vi "speed-test.vi"() -> ()   [LabVIEW 2020]
uses:
  <vilib>/Utility/Data Type/Type Definitions/Data Type.ctl
  <vilib>/Utility/Data Type/NI_Data Type.lvlib
panel:
  out "x-y":dbl
  out "Name":string
  out "number of dimensions":i32
  out "type":T1
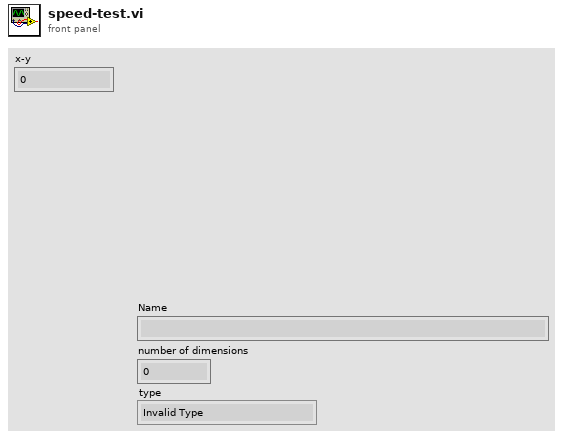
[diagram p1: front panel]
types:
  T1 = typedef "NI_Data Type.lvlib/Data Type.ctl" = enum8{"Invalid Type", "Void", "I8", "I16", "I32", "I64", "U8", "U16", "U32", "U64", "Single Float", "Double Float", "Extended Float", "Single Complex", "Double Complex", "Extended Complex", "Enum U8", "Enum U16", "Enum U32", "Enum U64", "Single Float With Unit", "Double Float With Unit", "Extended Float With Unit", "Single Complex with Unit", "Double Complex with Unit", "Extended Complex with Unit", "Boolean", "String", "Path", "Picture", "Tag", "Array", "Cluster", "Variant", "LV Variant", "Waveform", "Timestamp", "Digital Waveform", "Digital Data", "ExpressData", "Refnum", "External Data", "VI", "Poly VI", "LabVIEW Class Instance", "Fixed Point", "Set Collection", "Map Collection"}
  T2 = typedef "NI_Data Type.lvlib/Type Definition Info.ctl" = cluster{"Name":string, "Timestamp":u32}
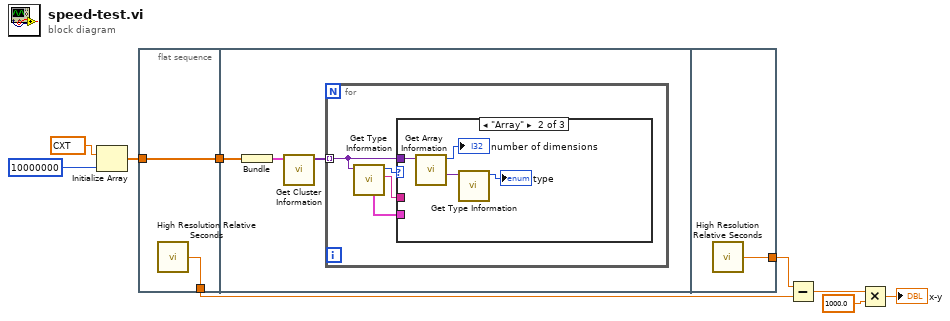
[diagram p0: block diagram]
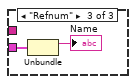
[diagram p3: hidden frame]
diagram:
  n1 = Initialize Array(cxt 0.0+0.0i ("element"), 10000000 ("dimension size")) -> (w7:cxt[])
  n2 = flat-sequence {
    tunnel: w7 -> [w11]
    tunnel: [w11] -> w6
    tunnel: [w10] -> w4
    tunnel: w6 -> [w13]
    tunnel: [w25] -> w5
    frame #0 {
      n3 = call <vilib>:"High Resolution Relative Seconds.vi"() -> ("relative seconds"=w10:dbl)
    }
    frame #1 {
      n4 = Bundle(w13) -> (w12:cluster{cxt[]})  [unwired: 1 in]
      n5 = call <vilib>:"Get Cluster Information.vi"("variant"=w12) -> ("cluster elements"=w14:variant[])  [unwired: 9 in, 1 out]
      n6 = for {
        tunnel: w14 -> [w15] mode=indexing
        n7 = call <vilib>:"Get Type Information.vi"("variant"=w15) -> ("name"=w16:string, "type"=w17:T1, "type definition info"=w18:T2)  [unwired: 6 in, 2 out]
        n8 = case shown="\"Array\"" w17 {
          tunnel: w18 -> [_ _ w24]
          tunnel: w16 -> [_ _ _]
          tunnel: w15 -> [_ w22 _]
          frame Default {
          }
          frame "Array" {
            n9 = call <vilib>:"Get Array Information.vi"("variant"=w22) -> ("array element data type"=w21:variant, "number of dimensions"=→"number of dimensions":i32)  [unwired: 7 in, 2 out]
            n10 = call <vilib>:"Get Type Information.vi"("variant"=w21) -> ("type"=→"type":T1)  [unwired: 6 in, 4 out]
          }
          frame "Refnum" {
            n11 = Unbundle(w24) -> ("Name"=→"Name":string)  [unwired: 1 out]
          }
        }
      }
    }
    frame #2 {
      n12 = call <vilib>:"High Resolution Relative Seconds.vi"() -> ("relative seconds"=w25:dbl)
    }
  }
  n13 = Subtract(x=w5, y=w4) -> (x-y=w3:dbl)
  n14 = Multiply(x=w3, y=1000.0) -> (x*y=→"x-y":dbl)
